vi "Pre-Arm.vi"(8 "error in (no error)":errorcluster, 11 "DAQmx Synthesizer in":refnum<class "DAQmx Synthesizer.lvclass">) -> (0 "error out":errorcluster, 3 "DAQmx Synthesizer out":refnum<class "DAQmx Synthesizer.lvclass">)   [LabVIEW 2021, in "DAQmx Synthesizer.lvclass"]
uses:
  DAQmx Synthesizer.lvclass
  DAQmx Digitizer/DAQmx Digitizer.lvclass
  DAQmx Synthesizer.lvclass/DAQmx Synthesizer.ctl
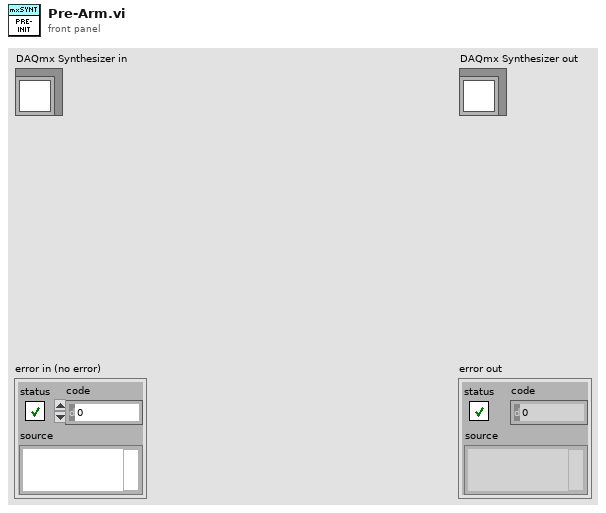
[diagram p1: front panel]
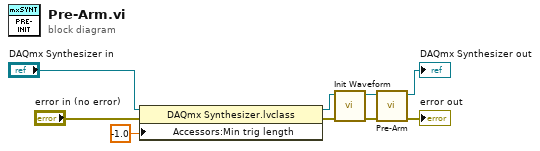
[diagram p0: block diagram]
diagram:
  n1 = property class="DAQmx Synthesizer.lvclass"(reference="DAQmx Synthesizer in", error in="error in (no error)", "Accessors:Min trig length"=-1.0 ("Min trig length")) -> (reference out=w2:refnum<class "DAQmx Synthesizer.lvclass">, error out=w4:errorcluster)
  n2 = call-dynamic "Init Waveform.vi"("error in (no error)"=w4, "DAQmx Synthesizer in"=w2) -> ("error out"=w5:errorcluster, "DAQmx Synthesizer out"=w7:refnum<class "DAQmx Synthesizer.lvclass">)  [unwired: 8 in]
  n3 = call-parent "Pre-Arm.vi"("error in (no error)"=w5, "DAQmx Digitizer in"=w7) -> ("error out"=→"error out":errorcluster, "DAQmx Digitizer out"=→"DAQmx Synthesizer out":refnum<class "DAQmx Synthesizer.lvclass">)  [unwired: 8 in]
